vi "rvd Braitenberg Map.vi"(9 "y Goal":i32, 10 "x Goal":i32, 11 "appended array":cluster{"X Value":dbl[], "Y Value":dbl[]}[](array[cluster])) -> (3 "Intensity Graph":dbl[][](graph))   [LabVIEW 2014]
panel:
  in  "reset":bool
  out "y Start":i32
  out "x Start":i32
  in  "Stop":bool
  # "X"
  # "Y"
  # "Start"
  # "Goal"
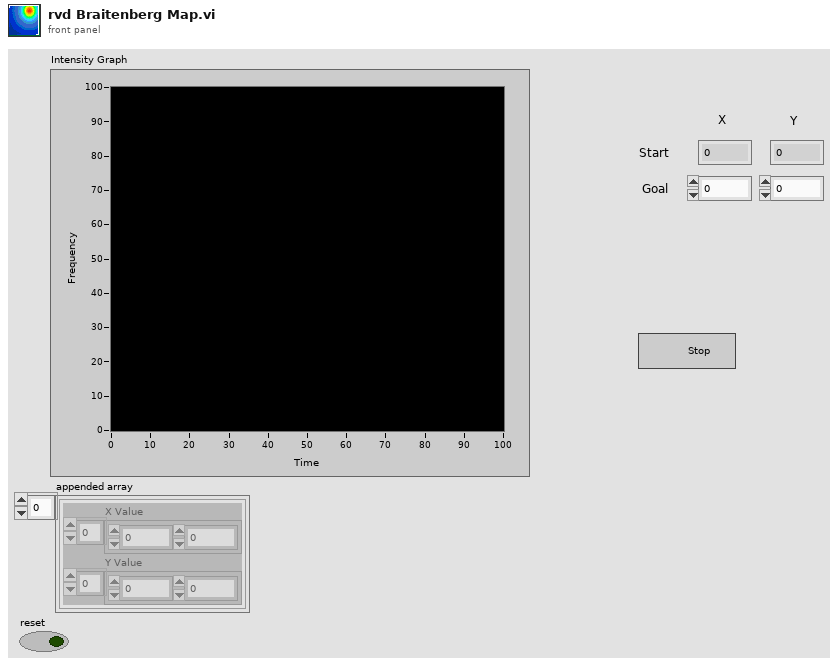
[diagram p1: front panel]
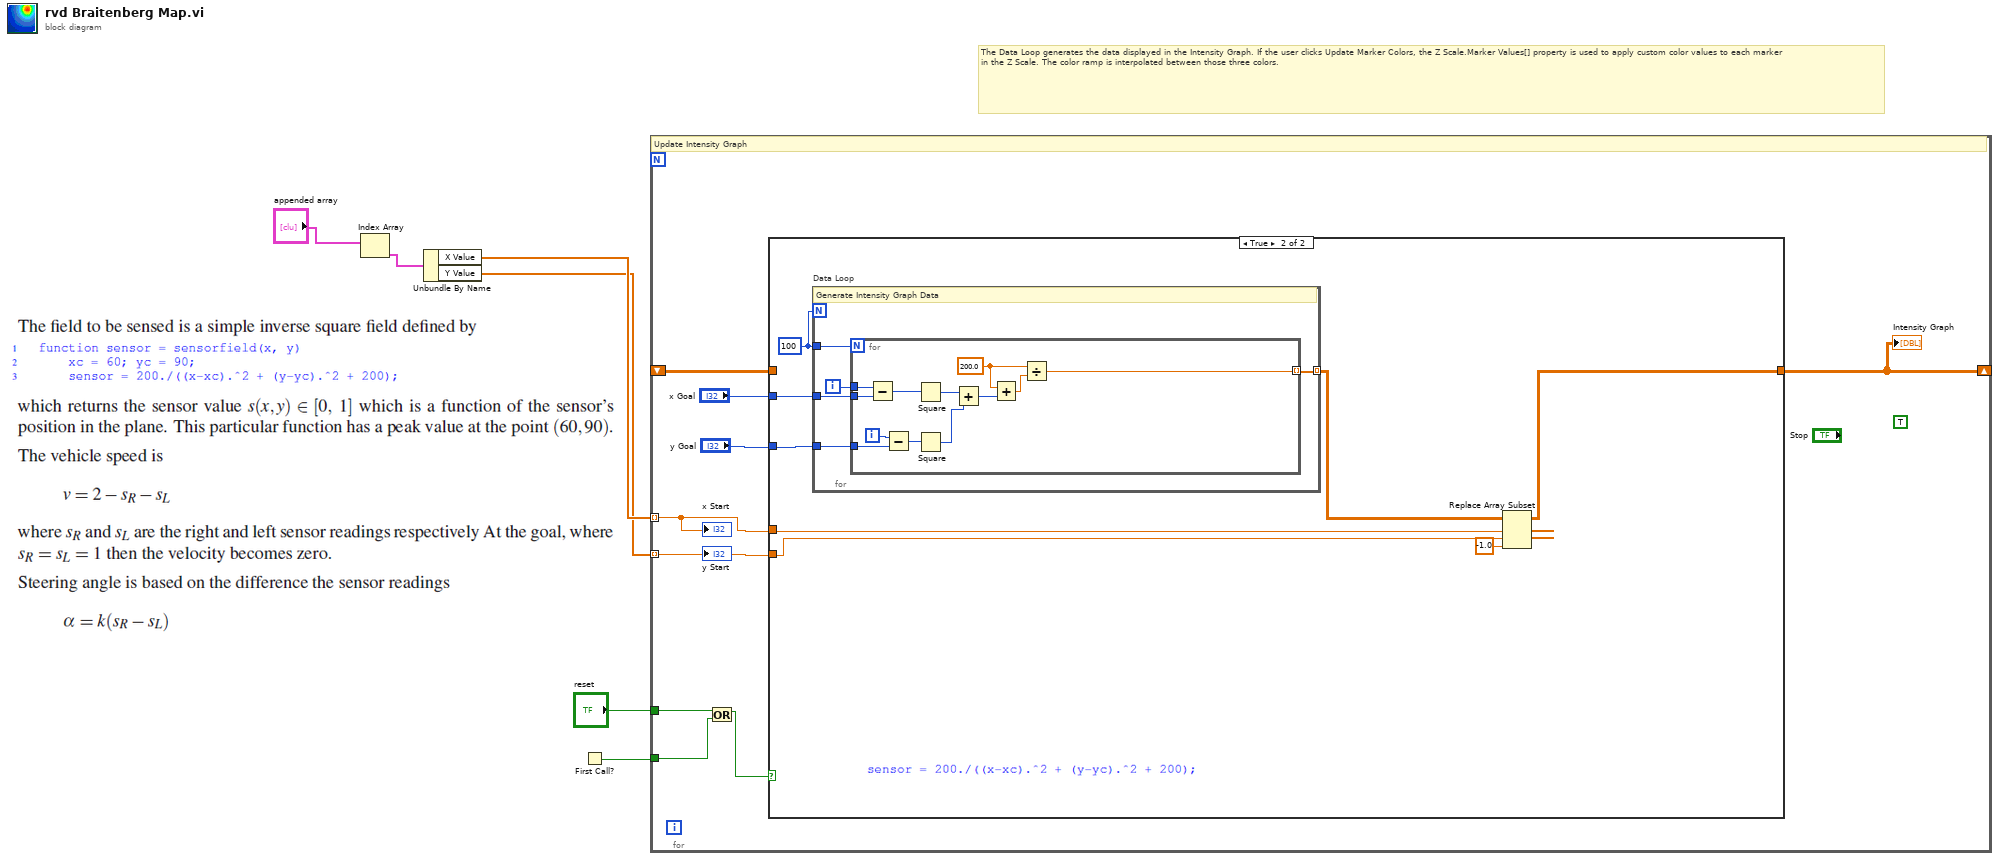
[diagram p0: block diagram]
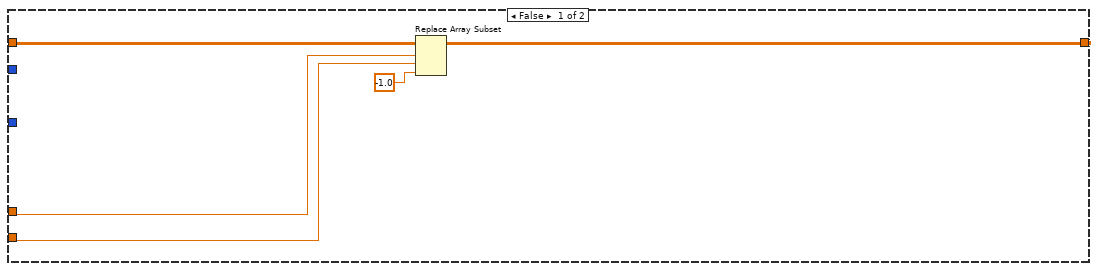
[diagram p2: hidden frame]
diagram:
  # "The Data Loop generates the data displayed in the Intensity Graph. If the user clicks Update Marker Colors, the Z Scale.Marker Values[] property is used to apply custom color values to each marker in the Z Scale. The color ramp is interpolated between those three colors."
  n1 = Index Array(array="appended array") -> (element=w5:cluster{"X Value":dbl[], "Y Value":dbl[]})  [unwired: 1 in]
  n2 = Unbundle By Name(w5) -> ("X Value"=w4:dbl[], "Y Value"=w3:dbl[])
  n3 = First Call?() -> (First Call?: T/F=w1:bool)
  n4 = for {
    shift-right: [w12] -> _
    shift-left: _ -> [w13]
    tunnel: w4 -> [w11] mode=indexing
    tunnel: w3 -> [w10] mode=indexing
    tunnel: "reset" -> [w8]
    tunnel: w1 -> [w7]
    (unwired) TRUE
    # "Update Intensity Graph"
    n5 = Or(x=w8, y=w7) -> (x .or. y?=w9:bool)
    n6 = case shown="True" w9 {
      tunnel: w10 -> [w17 w22]
      tunnel: w11 -> [w18 w23]
      tunnel: "y Goal" -> [_ w26]
      tunnel: "x Goal" -> [_ w27]
      tunnel: w13 -> [w20 _]
      tunnel: [w19 w24] -> w12
      frame False {
        n7 = Replace Array Subset(array=w20, new element=-1.0 ("new element/subarray"), index (row)=w18, index (col)=w17) -> (w19:dbl[][])
      }
      frame True {
        w28 = 100
        n8 = for "Data Loop" {
          N: w28 -> [_]
          tunnel: w28 -> [w33]
          tunnel: [w31] -> w25 mode=indexing
          tunnel: w27 -> [w30]
          tunnel: w26 -> [w29]
          i -> [w32]
          # "Generate Intensity Graph Data"
          n9 = for {
            N: w33 -> [_]
            tunnel: w32 -> [w39]
            tunnel: [w41] -> w31 mode=indexing
            tunnel: w30 -> [w35]
            tunnel: w29 -> [w34]
            i -> [w40]
            w37 = 200.0
            n10 = Subtract(x=w39, y=w35) -> (x-y=w45:i32)
            n11 = Subtract(x=w40, y=w34) -> (x-y=w44:i32)
            n12 = Square(x=w45) -> (x^2=w43:i32)
            n13 = Square(x=w44) -> (x^2=w42:i32)
            n14 = Add(x=w43, y=w42) -> (x+y=w38:i32)
            n15 = Add(x=w37, y=w38) -> (x+y=w36:dbl)
            n16 = Divide(x=w37, y=w36) -> (x/y=w41:dbl)
          }
        }
        n17 = Replace Array Subset(array=w25, new element=-1.0 ("new element/subarray"), index (row)=w23, index (col)=w22) -> (w24:dbl[][])
      }
    }
    "Intensity Graph" <- w12
    "x Start" <- w11
    "y Start" <- w10
  }
